vi "instance count allowed.vi"(8 "error in":errorcluster, 11 "alarms module configuration in":refnum<class "alarms module configuration.lvclass">) -> (0 "error out":errorcluster, 2 "instances allowed":i32, 3 "alarms module configuration out":refnum<class "alarms module configuration.lvclass">)   [LabVIEW 2013, in "alarms module configuration.lvclass"]
uses:
  alarms module configuration.lvclass
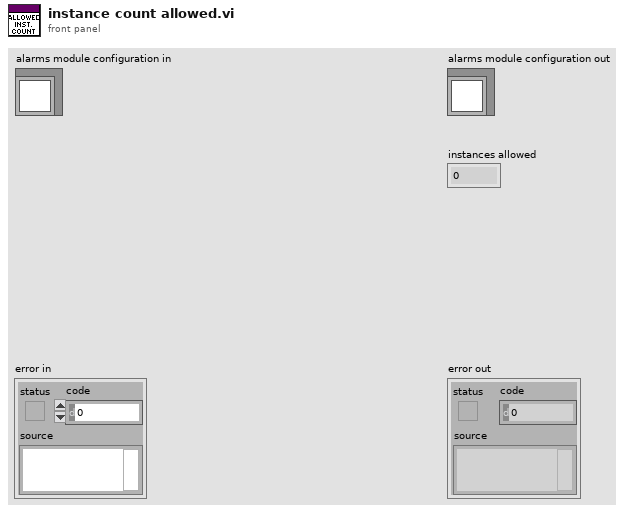
[diagram p1: front panel]
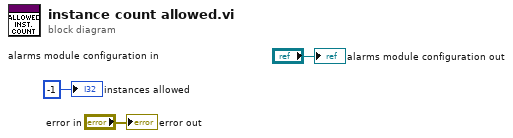
[diagram p0: block diagram]
diagram:
  "error out" <- "error in"
  "alarms module configuration out" <- "alarms module configuration in"
  "instances allowed" <- -1 ("instances allowed")
